vi "InitFromXML.vi"(8 "error in (no error)":errorcluster, 10 "XML":string, 11 "ProjectWizardClickableText in":refnum<class "ProjectWizardClickableText.lvclass">) -> (0 "error out":errorcluster, 3 "ProjectWizardClickableText out":refnum<class "ProjectWizardClickableText.lvclass">)   [LabVIEW 2009, in "NavScreen.lvlib" / "ProjectWizardClickableText.lvclass"]
uses:
  ProjectWizardClickableText.lvclass
  ClickableText/ClickableText.lvclass
  ProjectWizardClickableText.lvclass/ProjectWizardClickableText.ctl
  NavScreen.lvlib
  ProjectWizard/ProjectWizard.lvclass
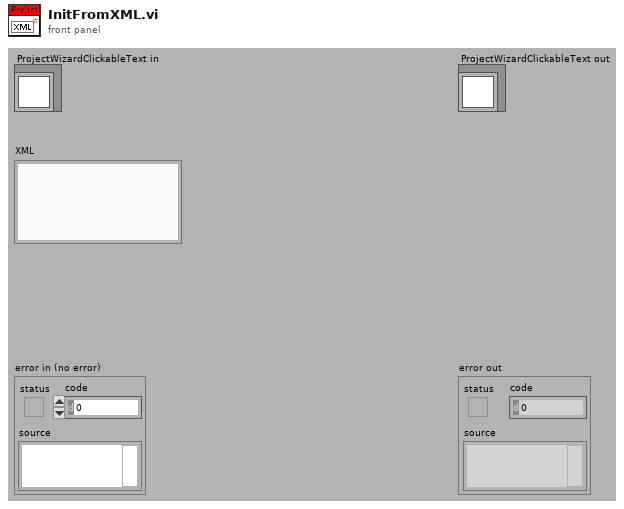
[diagram p1: front panel]
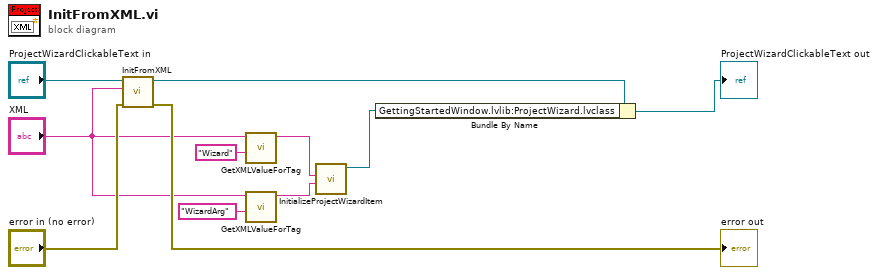
[diagram p0: block diagram]
diagram:
  n1 = call-parent "InitFromXML.vi"("error in (no error)"="error in (no error)", "XML"="XML", "ClickableText in"="ProjectWizardClickableText in") -> ("error out"=→"error out":errorcluster, "ClickableText out"=w3:refnum<class "ProjectWizardClickableText.lvclass">)  [unwired: 7 in]
  n2 = call "GetXMLValueForTag.vi"("tag"="Wizard", "XML"="XML") -> ("value"=w5:string)  [unwired: 8 in, 1 out]
  n3 = call "GetXMLValueForTag.vi"("tag"="WizardArg", "XML"="XML") -> ("value"=w4:string)  [unwired: 8 in, 1 out]
  n4 = call "InitializeProjectWizardItem.vi"("wizard argument"=w4, "wizard"=w5) -> ("ProjectWizard out"=w1:refnum<class "ProjectWizard.lvclass">)  [unwired: 8 in, 1 out]
  n5 = Bundle By Name(cluster=w3, "GettingStartedWindow.lvlib:ProjectWizard.lvclass"=w1) -> (→"ProjectWizardClickableText out":refnum<class "ProjectWizardClickableText.lvclass">)
